vi "reshapeArray.vi"(7 "reshapeInfo":T2, 9 "element":T1, 11 "z":dbl[][](array[numeric])) -> (3 "reshaped array":dbl[](array[numeric]))   [LabVIEW 2013]
uses:
  reshapeINfo_TypDef.ctl
  emptyArray_TYpDEf.ctl
  emptyArrayCamX_TypDef.ctl
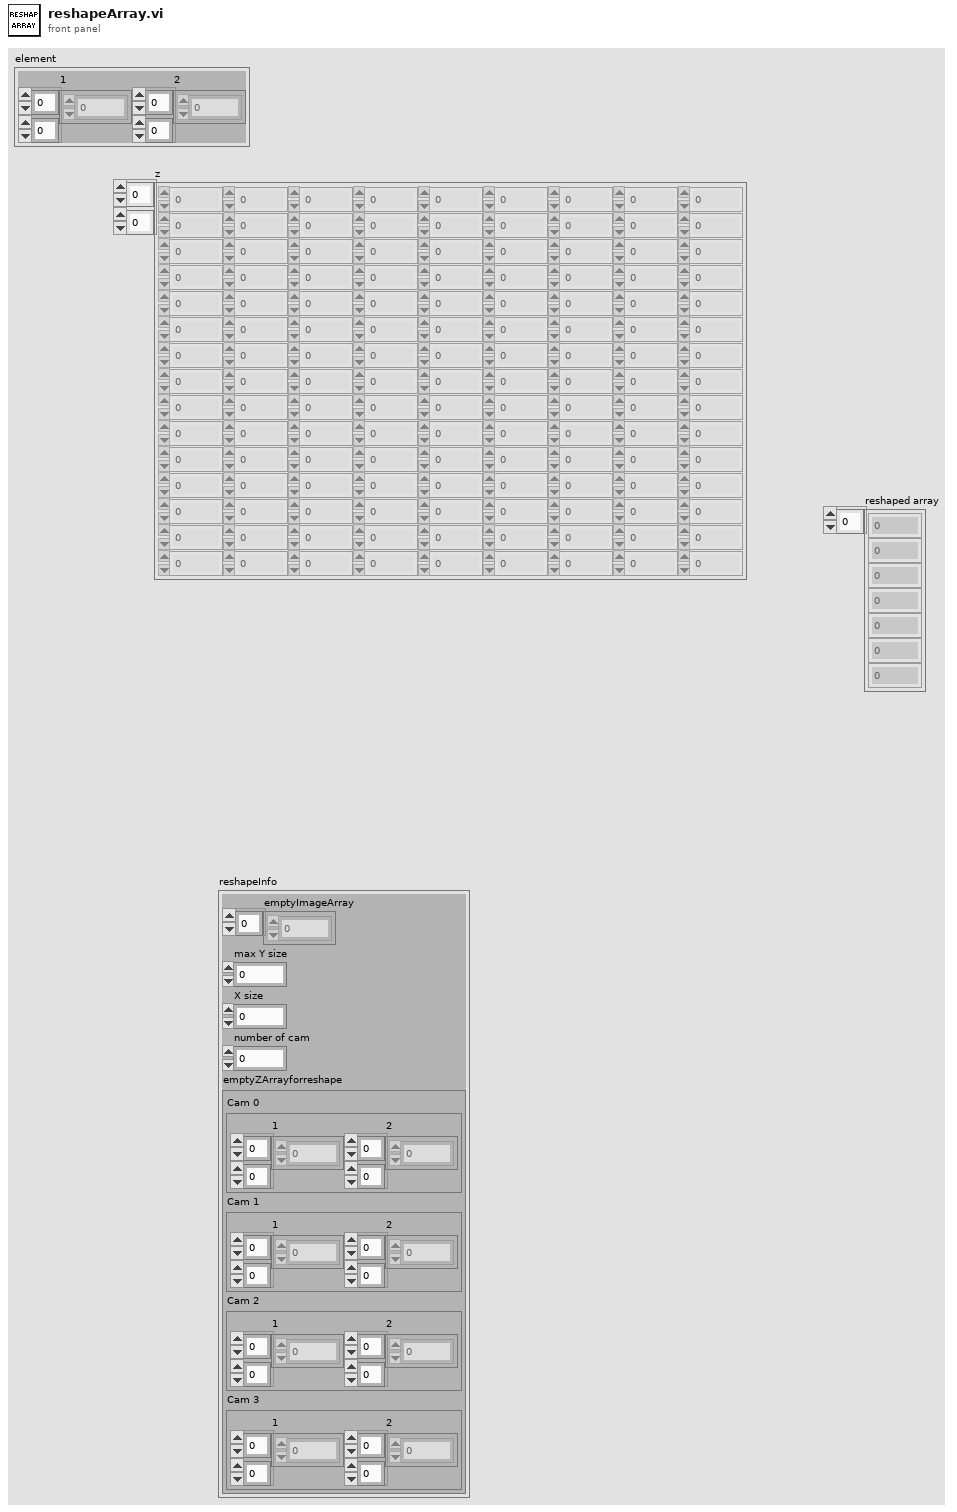
[diagram p1: front panel]
types:
  T1 = typedef "emptyArrayCamX_TypDef.ctl" = cluster{"1":dbl[][], "2":dbl[][]}
  T2 = typedef "reshapeINfo_TypDef.ctl" = cluster{"emptyImageArray":dbl[], "max Y size":i32, "X size":i32, "number of cam":i32, "emptyZArrayforreshape":T3}
  T3 = typedef "emptyArray_TYpDEf.ctl" = cluster{"Cam 0":T1, "Cam 1":T1, "Cam 2":T1, "Cam 3":T1}
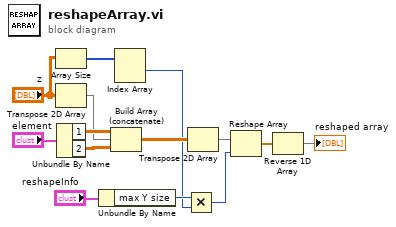
[diagram p0: block diagram]
diagram:
  n1 = Array Size(array="z") -> (size(s)=w7:i32[])
  n2 = Transpose 2D Array(2D array="z") -> (transposed array=w5:dbl[][])
  n3 = Unbundle By Name("element") -> ("1"=w10:dbl[][], "2"=w9:dbl[][])
  n4 = Unbundle By Name("reshapeInfo") -> ("max Y size"=w12:i32)
  n5 = Build Array (concatenate)(w10, w5, w9) -> (w4:dbl[][])
  n6 = Index Array(array=w7) -> (element #1=w1:i32)  [unwired: 2 in, 1 out]
  n7 = Multiply(x=w12, y=w1) -> (x*y=w2:i32)
  n8 = Transpose 2D Array(2D array=w4) -> (transposed array=w6:dbl[][])
  n9 = Reshape Array(w6, w2) -> (w13:dbl[])
  n10 = Reverse 1D Array(array=w13) -> (reversed array=→"reshaped array":dbl[])
